vi "Cog Detector.vi"(0 "Cog Limits:":i32[](array[numeric])=[0, 0, 0, 0, 0, 0], 5 "Cogs IN":i32[](array[numeric]), 7 "Counters IN":i32[](array[numeric]), 9 "Started":bool[](array[boolean]), 11 "Pump Present":bool[](array[boolean]), 12 "Flow":dbl[](array[numeric])=[0.0, 0.0, 0.0, 0.125, 0.0625, 0.0625] caption="Flow\n(L/H)" format="%#.0f", 13 "Run Profile":bool) -> (4 "Cogs OUT":i32[](array[numeric]), 8 "Cog Alarm":bool, 15 "Counters OUT":i32[](array[numeric]))   [LabVIEW 2019]
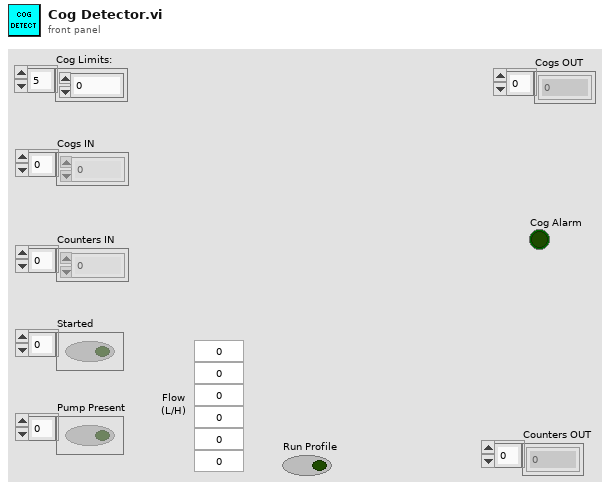
[diagram p1: front panel]
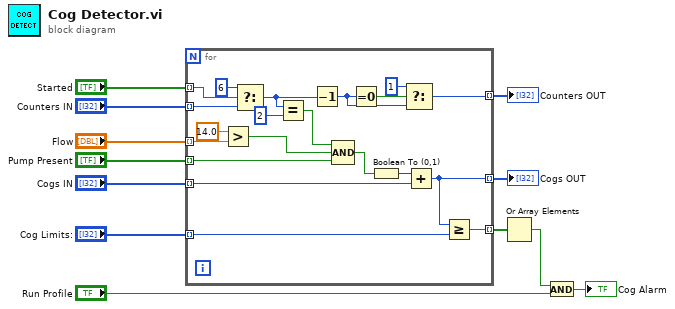
[diagram p0: block diagram]
diagram:
  n1 = for {
    tunnel: "Pump Present" -> [w20] mode=indexing
    tunnel: "Started" -> [w29] mode=indexing
    tunnel: "Counters IN" -> [w30] mode=indexing
    tunnel: "Cogs IN" -> [w32] mode=indexing
    tunnel: [w15] -> w8 mode=indexing
    tunnel: "Flow" -> [w17] mode=indexing
    tunnel: [w24] -> w6 mode=indexing
    tunnel: "Cog Limits:" -> [w14] mode=indexing
    tunnel: [w13] -> w4 mode=indexing
    n2 = Greater?(x=14.0 ("y"), y=w17) -> (0:w19:bool)
    n3 = Select(t=6, s=w29, f=w30) -> (s? t:f=w22:i32)
    n4 = Equal?(x=w22, y=2 ("t")) -> (x = y?=w21:bool)
    n5 = Decrement(x=w22) -> (x-1=w26:i32)
    n6 = Compound Arithmetic op=AND(w21, w19, w20) -> (w18:bool)
    n7 = Equal To 0?(x=w26) -> (x = 0?=w27:bool)
    n8 = Boolean To (0,1)(Boolean=w18) -> (0, 1=w31:i16)
    n9 = Select(t=1, s=w27, f=w26) -> (s? t:f=w24:i32)
    n10 = Add(x=w31, y=w32) -> (x+y=w15:i32)
    n11 = Greater Or Equal?(x=w15, y=w14) -> (x >= y?=w13:bool)
  }
  "Counters OUT" <- w6
  "Cogs OUT" <- w8
  n12 = Or Array Elements(Boolean array=w4) -> (logical OR=w2:bool)
  n13 = And(x=w2, y="Run Profile") -> (x .and. y?=→"Cog Alarm":bool)
